vi "ReadFromDS.vi"(3 "DS Server\nIP Address":refnum<k13>) -> (0 "error out":errorcluster, 1 "Data Received":string)   [LabVIEW 2012]
doc: "This example illustrates using datasocket for reading in a waveform. \n \nIt works with http, ftp,and local files, as well as with live data. \n\nTo use with static files, select one of the URLs beginning with file, ftp, or http listed at the bottom of the front panel, and enter it into the text box. Then start the VI. \n \nTo use it with live data, start the DataSocket Server from the Start menu and run the LVDSWriter example. Then select the same URL (dstp://localhost/wave) for this example and press the connect button. \n \nThe Writer, Server, and Reader can all be on the same machine or different machines. The Writer's and Reader's URL should point to the machine that the DataSocket Server is on."
panel:
  out "Status":string
  in  "stop":bool
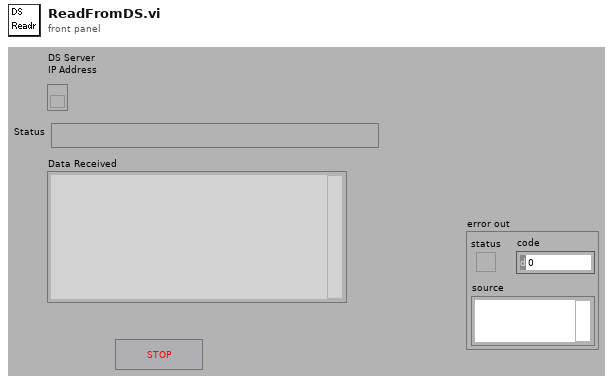
[diagram p1: front panel]
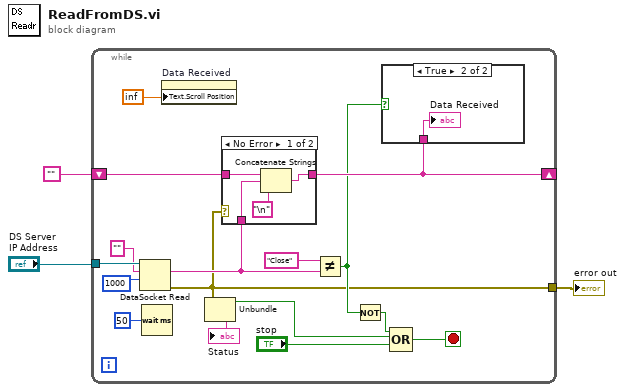
[diagram p0: block diagram]
diagram:
  n1 = while {
    tunnel: [w4] -> w1
    tunnel: "DS Server\nIP Address" -> [w19]
    shift-right: [w11] -> _
    shift-left: "" -> [w12]
    stop <- w5 stop-if-true
    n2 = DataSocket Read(9:1000 ("ms timeout (10000)"), 10:"", 11:w19) -> (0:w4:errorcluster, 2:w10:string)  [unwired: 1 in, 6 out]
    n3 = Wait (ms)(milliseconds to wait=u32 50) -> ()  [unwired: 1 out]
    n4 = property on="Data Received" class="Str"("Text.Scroll Position"=inf) -> ()  [unwired: 2 in, 2 out]
    n5 = Unbundle(w4) -> ("status"=w8:bool, "source"=→"Status":string)  [unwired: 1 out]
    n6 = case shown="No Error" w4 {
      tunnel: w12 -> [w24 w25]
      tunnel: w10 -> [w23 _]
      tunnel: [w21 w25] -> w11
      frame No Error {
        n7 = Concatenate Strings(w24, w23, "\n") -> (w21:string)
      }
      frame Error {
      }
    }
    n8 = Not Equal?(x="Close", y=w10) -> (x != y?=w9:bool)
    n9 = Not(x=w9) -> (.not. x?=w6:bool)
    n10 = case shown="True" w9 {
      tunnel: w11 -> [_ w20]
      frame False {
      }
      frame True {
        "Data Received" <- w20
      }
    }
    n11 = Compound Arithmetic op=OR(w6, w8, "stop") -> (w5:bool)
  }
  "error out" <- w1
